vi "GetLatestDataPackage.vi"(0 "SmartScope in":refnum<k24>) -> (1 "SmartScope out":refnum<k24>, 2 "DataPackage":refnum<k24>)   [LabVIEW 2013]
uses:
  C:/Program Files (x86)/LabNation/SmartScope/DeviceInterface.dll
  Program Files (x86)/LabNation/SmartScope/DeviceInterface.dll
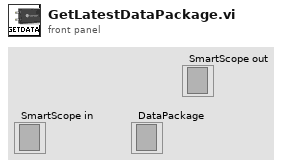
[diagram p1: front panel]
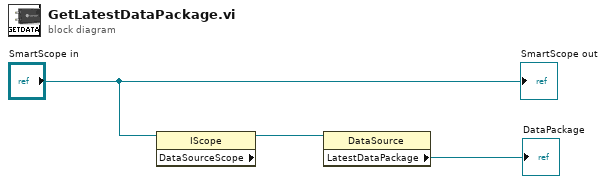
[diagram p0: block diagram]
diagram:
  n1 = property class="IScope"(reference="SmartScope in") -> ("DataSourceScope"=w3:refnum<k24>)  [unwired: 1 in, 2 out]
  n2 = property class="DataSource"(reference=w3) -> ("LatestDataPackage"=→"DataPackage":refnum<k24>)  [unwired: 1 in, 2 out]
  "SmartScope out" <- "SmartScope in"
